vi "Create Subsystem.vi"(8 "error in (no error)":errorcluster, 9 "Subsystem I/O Attributes":T2[](array[typedef]), 10 "Subsystem":T1={"Name"="Control1", "Root URL"=""}, 11 "System Name":string) -> (0 "error out":errorcluster)   [LabVIEW 2024]
doc: "Creates a subsystem in the shared variable engine."
uses:
  Controls/Server/Subsystem IO Attributes.ctl
  Controls/Server/Subsystem IO Logging Attributes.ctl
  Controls/Server/Subsystem IO Alarm Attributes.ctl
  Controls/Server/Subsystem Configuration.ctl
  <vilib>/lvdsc/variables/internal/Configure Alarming (Shared Variable, Enable Alarming).vi
  <vilib>/lvdsc/variables/internal/Configure Alarming (Shared Variable, Bad Status).vi
  <vilib>/lvdsc/variables/internal/Configure Alarming (Shared Variable, Boolean).vi
  <vilib>/lvdsc/variables/internal/Configure Alarming (Shared Variable, Numeric).vi
  <vilib>/lvdsc/NI_DSC.lvlib
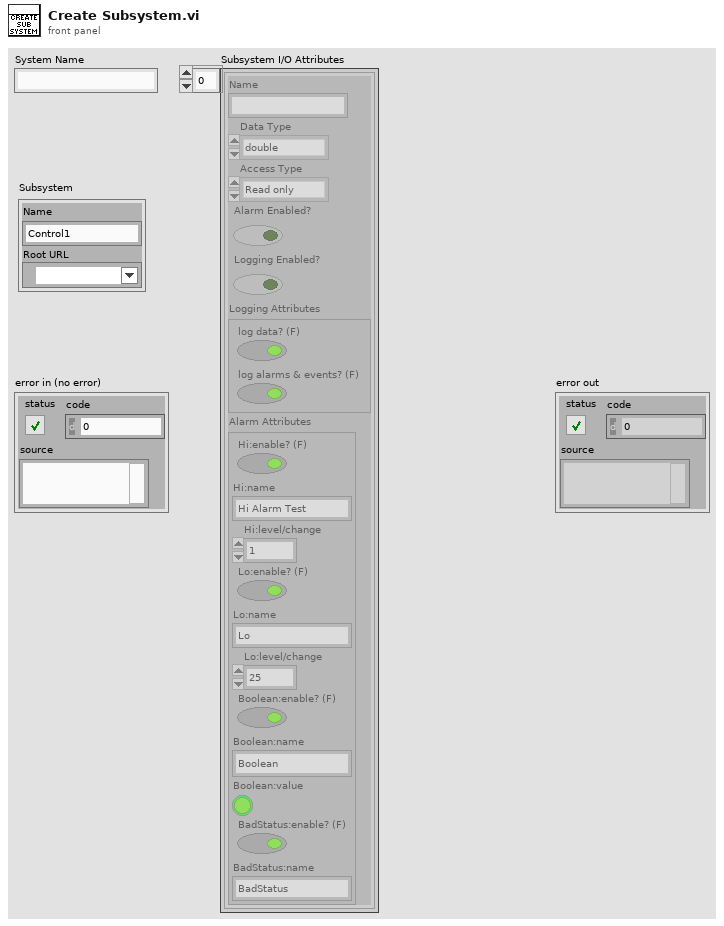
[diagram p1: front panel]
types:
  T1 = typedef "Subsystem Configuration.ctl" = cluster{"Name":string, "Root URL":refnum<k21>}
  T2 = typedef "Subsystem IO Attributes.ctl" = cluster{"Name":string, "Data Type":enum32{"u32BitField", "bool", "double", "string", "int8", "uint8", "int16", "uint16", "int32", "uint32", "int64", "uint64", "single", "double waveform", "int16 waveform", "array of boolean", "array of int8", "array of uint8", "array of int16", "array of uint16", "array of int32", "array of uint32", "array of int64", "array of uint64", "array of single", "array of double", "array of double waveform", "array of int16 waveform", "array of string", "variant", "timestamp", "fixed point", "custom"}, "Access Type":enum32{"Read only", "Write only", "Read/write"}, "Alarm Enabled?":bool, "Logging Enabled?":bool, "Logging Attributes":T3, "Alarm Attributes":T4}
  T3 = typedef "Subsystem IO Logging Attributes.ctl" = cluster{"log data? (F)":bool, "log alarms & events? (F)":bool}
  T4 = typedef "Subsystem IO Alarm Attributes.ctl" = cluster{"Hi:enable? (F)":bool, "Hi:name":string, "Hi:level/change":dbl, "Lo:enable? (F)":bool, "Lo:name":string, "Lo:level/change":dbl, "Boolean:enable? (F)":bool, "Boolean:name":string, "Boolean:value":bool, "BadStatus:enable? (F)":bool, "BadStatus:name":string}
  T5 = cluster{"enable? (F)":bool, "data type (deprecated)":enum32{"U32 Bit Field", "Boolean", "Double", "String"}, "log data? (F)":bool, "log alarms & events? (F)":bool, "value resolution (for Float variables only)":dbl, "value deadband (for Float variables only)":dbl, "string logging format (for String variables only)":u32}
  T6 = cluster{"use binding? (F)":bool, "URL":string, "access type":enum32{"Read only", "Write only", "Read/write"}, "buffer size":u32, "use buffering? (F)":bool, "single writer? (F)":bool}
  T7 = cluster{"enable? (F)":bool, "name":string, "priority":u32, "ack type":enum16{"Auto", "User", "None"}, "area":string, "description":string, "log? (T)":bool}
  T8 = cluster{"enable? (F)":bool, "name":string, "alarm on":bool, "priority":u32, "ack type":enum16{"Auto", "User", "None"}, "area":string, "description":string, "log? (T)":bool}
  T9 = cluster{"enable? (F)":bool, "name":string, "alarm type":enum16{"HI_HI", "HI", "LO", "LO_LO"}, "level/change":dbl, "deadband/time":dbl, "priority":u32, "ack type":enum16{"Auto", "User", "None"}, "area":string, "description":string, "log? (T)":bool}
  T10 = enum32{"u32BitField", "bool", "double", "string", "int8", "uint8", "int16", "uint16", "int32", "uint32", "int64", "uint64", "single", "double waveform", "int16 waveform", "array of boolean", "array of int8", "array of uint8", "array of int16", "array of uint16", "array of int32", "array of uint32", "array of int64", "array of uint64", "array of single", "array of double", "array of double waveform", "array of int16 waveform", "array of string", "variant", "timestamp", "fixed point", "custom"}
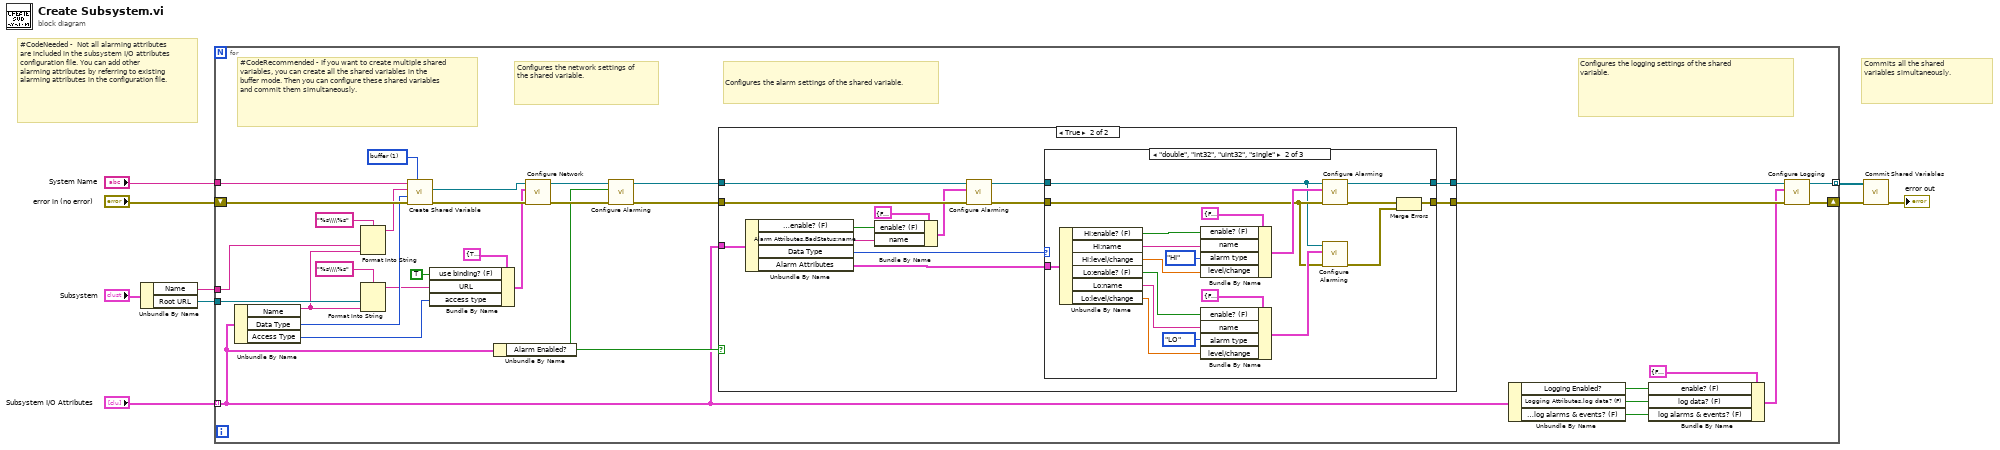
[diagram p0: block diagram]
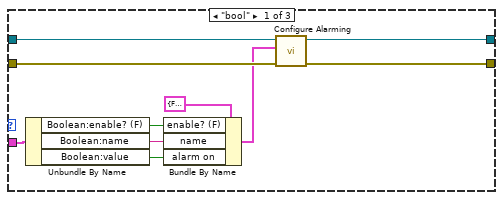
[diagram p3: hidden frame]
diagram:
  # "#CodeNeeded -  Not all alarming attributes are included in the subsystem I/O attributes configuration file. You can add other alarming attributes by referring to existing alarming attributes in the configuration file."
  # "Commits all the shared variables simultaneously."
  n1 = Unbundle By Name("Subsystem") -> ("Name"=w6:string, "Root URL"=w7:refnum<k21>)
  n2 = for {
    tunnel: "Subsystem I/O Attributes" -> [w22] mode=indexing
    tunnel: w7 -> [w32]
    tunnel: w6 -> [w41]
    shift-right: [w18] -> w4
    shift-left: "error in (no error)" -> [w39]
    tunnel: [w13] -> w2 mode=indexing
    tunnel: "System Name" -> [w10]
    w12 = u16 1 items=["commit", "buffer"] ("set mode")
    # "Configures the alarm settings of the shared variable."
    # "#CodeRecommended - If you want to create multiple shared variables, you can create all the shared variables in the buffer mode. Then you can configure these shared variables and commit them simultaneously."
    # "Configures the logging settings of the shared variable."
    # "Configures the network settings of the shared variable."
    n3 = Unbundle By Name(w22) -> ("Name"=w31:string, "Data Type"=w35:T10, "Access Type"=w11:enum32{"Read only", "Write only", "Read/write"})
    n4 = Format Into String(format string="%s\\\\%s", w41, w31) -> (resulting string=w38:string)  [unwired: 2 in, 1 out]
    n5 = Format Into String(format string="%s\\\\%s", w32, w31) -> (resulting string=w30:string)  [unwired: 2 in, 1 out]
    n6 = call <vilib>:"Create Shared Variable.vi"("set mode"=w12, "error in (no error)"=w39, "data type"=w35, "shared variable name"=w38, "process name"=w10) -> ("error out"=w37:errorcluster, "shared variable"=w36:refnum<k21>)  [unwired: 4 in, 1 out]
    n7 = Bundle By Name(cluster=T6 {"use binding? (F)"=TRUE, "URL"="", "access type"=enum."Read/write", "buffer size"=50, "use buffering? (F)"=FALSE, "single writer? (F)"=FALSE} ("network settings"), "use binding? (F)"=TRUE, "URL"=w30, "access type"=w11) -> (w29:T6)
    n8 = Unbundle By Name(w22) -> ("Alarm Enabled?"=w23:bool)
    n9 = call <vilib>:"Configure Network.vi"("error in (no error)"=w37, "network settings"=w29, "variable reference in"=w36) -> ("error out"=w27:errorcluster, "variable reference out"=w28:refnum<k21>)  [unwired: 7 in]
    n10 = call-poly <vilib>:"Configure Alarming.vi"("error in (no error)"=w27, "enable? (F)"=w23, "variable reference in"=w28) -> ("error out"=w26:errorcluster, "variable reference out"=w25:refnum<k21>)  [unwired: 7 in]
    n11 = case shown="True" w23 {
      tunnel: w26 -> [w43 w55]
      tunnel: [w43 w45] -> w19
      tunnel: w25 -> [w42 w56]
      tunnel: [w42 w44] -> w17
      tunnel: w22 -> [_ w54]
      frame False {
      }
      frame True {
        n12 = Unbundle By Name(w54) -> ("Alarm Attributes.BadStatus:enable? (F)"=w52:bool, "Alarm Attributes.BadStatus:name"=w51:string, "Data Type"=w49:T10, "Alarm Attributes"=w46:T4)
        n13 = Bundle By Name(cluster=T7 {"enable? (F)"=FALSE, "name"="Status", "priority"=1, "ack type"=enum."Auto", "area"="", "description"="", "log? (T)"=TRUE} ("bad status alarm settings"), "enable? (F)"=w52, "name"=w51) -> (w50:T7)
        n14 = call-poly <vilib>:"Configure Alarming.vi"("error in (no error)"=w55, "bad status alarm settings"=w50, "variable reference in"=w56) -> ("error out"=w48:errorcluster, "variable reference out"=w47:refnum<k21>)  [unwired: 7 in]
        n15 = case shown="\"double\", \"int32\", \"uint32\", \"single\"" w49 {
          tunnel: w48 -> [w65 w71 w86]
          tunnel: w47 -> [w66 w67 w87]
          tunnel: w46 -> [w62 w85 _]
          tunnel: [w58 w69 w86] -> w45
          tunnel: [w57 w72 w87] -> w44
          frame "bool" {
            n16 = Unbundle By Name(w62) -> ("Boolean:enable? (F)"=w61:bool, "Boolean:name"=w60:string, "Boolean:value"=w59:bool)
            n17 = Bundle By Name(cluster=T8 {"enable? (F)"=FALSE, "name"="Boolean", "alarm on"=TRUE, "priority"=1, "ack type"=enum."Auto", "area"="", "description"="", "log? (T)"=TRUE} ("Boolean alarm settings"), "enable? (F)"=w61, "name"=w60, "alarm on"=w59) -> (w63:T8)
            n18 = call-poly <vilib>:"Configure Alarming.vi"("error in (no error)"=w65, "Boolean alarm settings"=w63, "variable reference in"=w66) -> ("error out"=w58:errorcluster, "variable reference out"=w57:refnum<k21>)  [unwired: 7 in]
          }
          frame "double", "int32", "uint32", "single" {
            n19 = Unbundle By Name(w85) -> ("Hi:enable? (F)"=w79:bool, "Hi:name"=w80:string, "Hi:level/change"=w82:dbl, "Lo:enable? (F)"=w78:bool, "Lo:name"=w77:string, "Lo:level/change"=w75:dbl)
            n20 = Bundle By Name(cluster=T9 {"enable? (F)"=FALSE, "name"="HiHi", "alarm type"=enum."HI_HI", "level/change"=90.0, "deadband/time"=1.0, "priority"=1, "ack type"=enum."Auto", "area"="", "description"="", "log? (T)"=TRUE} ("numeric alarm settings"), "enable? (F)"=w79, "name"=w80, "alarm type"=enum16{"HI_HI", "HI", "LO", "LO_LO"}."HI", "level/change"=w82) -> (w73:T9)
            n21 = Bundle By Name(cluster=T9 {"enable? (F)"=FALSE, "name"="HiHi", "alarm type"=enum."HI_HI", "level/change"=90.0, "deadband/time"=1.0, "priority"=1, "ack type"=enum."Auto", "area"="", "description"="", "log? (T)"=TRUE} ("numeric alarm settings"), "enable? (F)"=w78, "name"=w77, "alarm type"=enum16{"HI_HI", "HI", "LO", "LO_LO"}."LO", "level/change"=w75) -> (w74:T9)
            n22 = call-poly <vilib>:"Configure Alarming.vi"("error in (no error)"=w71, "numeric alarm settings"=w73, "variable reference in"=w67) -> ("error out"=w70:errorcluster, "variable reference out"=w72:refnum<k21>)  [unwired: 7 in]
            n23 = call-poly <vilib>:"Configure Alarming.vi"("error in (no error)"=w71, "numeric alarm settings"=w74, "variable reference in"=w67) -> ("error out"=w68:errorcluster)  [unwired: 7 in, 1 out]
            n24 = Merge Errors(w70, w68) -> (w69:errorcluster)
          }
          frame Default {
          }
        }
      }
    }
    n25 = Unbundle By Name(w22) -> ("Logging Enabled?"=w20:bool, "Logging Attributes.log data? (F)"=w16:bool, "Logging Attributes.log alarms & events? (F)"=w15:bool)
    n26 = Bundle By Name(cluster=T5 {"enable? (F)"=FALSE, "data type (deprecated)"=enum."U32 Bit Field", "log data? (F)"=FALSE, "log alarms & events? (F)"=FALSE, "value resolution (for Float variables only)"=0.01, "value deadband (for Float variables only)"=0.01, "string logging format (for String variables only)"=0} ("logging settings"), "enable? (F)"=w20, "log data? (F)"=w16, "log alarms & events? (F)"=w15) -> (w14:T5)
    n27 = call <vilib>:"Configure Logging.vi"("error in (no error)"=w19, "logging settings"=w14, "variable reference in"=w17) -> ("error out"=w18:errorcluster, "variable reference out"=w13:refnum<k21>)  [unwired: 7 in]
  }
  n28 = call <vilib>:"Commit Shared Variables.vi"("error in (no error)"=w4, "shared variables"=w2) -> ("error out"=→"error out":errorcluster)  [unwired: 9 out]
